vi "PId.vi"(8 "Ts [s]":dbl, 9 "PI Parameters":cluster{"Kp":dbl, "Ti [s]":dbl}, 10 "Reference Value":dbl, 11 "Process Value [°C]":dbl) -> (2 "Control Value (u)":dbl)   [LabVIEW 2025]
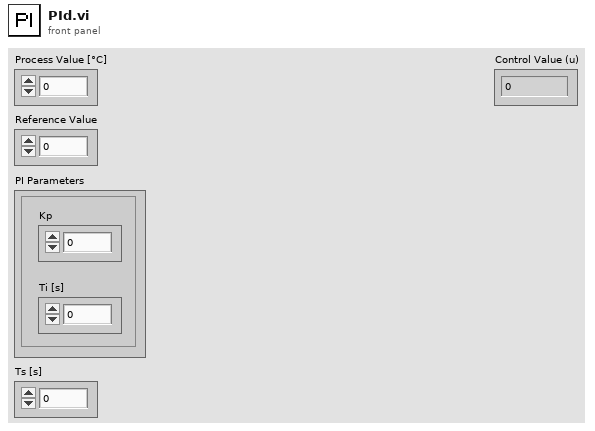
[diagram p1: front panel]
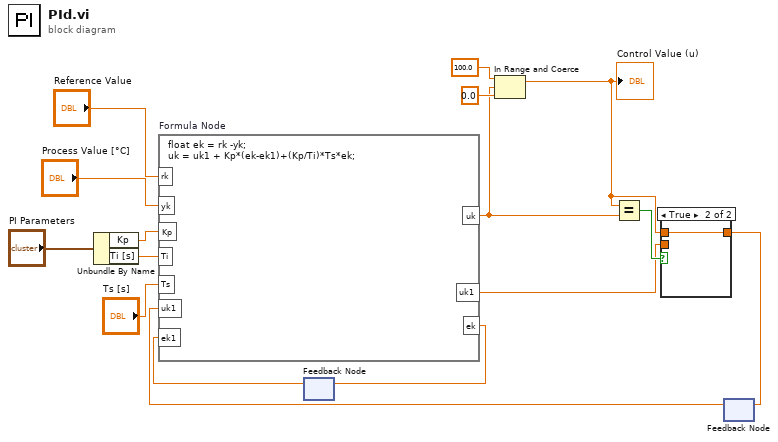
[diagram p0: block diagram]
diagram:
  n1 = Unbundle By Name("PI Parameters") -> ("Kp"=w13:dbl, "Ti [s]"=w12:dbl)
  n2 = feedback #1() -> (w5:dbl)  [unwired: 1 in]
  n3 = feedback #2() -> (w6:dbl)  [unwired: 1 in]
  n4 = formula code="float ek = rk -yk;\nuk = uk1 + Kp*(ek-ek1)+(Kp/Ti)*Ts*ek;"("rk"="Reference Value", "yk"="Process Value [°C]", "Kp"=w13, "Ti"=w12, "Ts"="Ts [s]", "uk1"=w6, "ek1"=w5) -> ("uk"=w4:dbl, "ek"=w3:dbl, "uk1"=w2:dbl)
  n5 = feedback-in #1(w3) -> ()
  n6 = In Range and Coerce(upper limit=100.0, x=w4, lower limit=0.0) -> (coerced(x)=w1:dbl)  [unwired: 1 out]
  "Control Value (u)" <- w1
  n7 = Equal?(x=w1, y=w4) -> (x = y?=w8:bool)
  n8 = case shown="True" w8 {
    tunnel: w1 -> [_ w18]
    tunnel: [w17 w18] -> w7
    tunnel: w2 -> [w17 _]
    frame False {
    }
    frame True {
    }
  }
  n9 = feedback-in #2(w7) -> ()
